vi "1 port_Parametric Calculations_MultiTest.vi"(0 "Port Measurements":T1, 2 "Specific Voltages":dbl[](array[numeric])=[32.0, 36.0], 11 "Error In":errorcluster) -> (4 "One_port_Parametric Calculated Values":T4, 15 "Error Out":errorcluster)   [LabVIEW 2013]
uses:
  Controls/Port Measurements.ctl
  Controls/1 port_Parametric Calculated Values.ctl
  Controls/Port Capacitance Parametric Calculations.ctl
  Controls/Port Voltage Parametric Calculations.ctl
  Controls/Port Resistance Parametric Calculations.ctl
  Controls/Resistance Array Calculated Values.ctl
  Controls/Individual User Inputs_MultiTest.ctl
  Controls/Test Selection.ctl
panel:
  in  "Tab Control":enum32{"Inputs", "Outputs"}(tab)
  in  "Selected Exp Settings":T2={"Floor_Sweep_Stop_V"=36.0, "Resistance Threshold"=1.0, "Floor_Sweep_Start_V"=36.0, "Floor_Sweep_Step_V"=1.0, "Roof_Sweep_Stop_V"=36.0, "Roof_Sweep_Start_V"=36.0, "Roof_Sweep_Step_V"=1.0, "Experiment Name"="", "Meas_Type"=[0, 2, 4]}
  # "Calculation Settings"
  # "Test Settings"
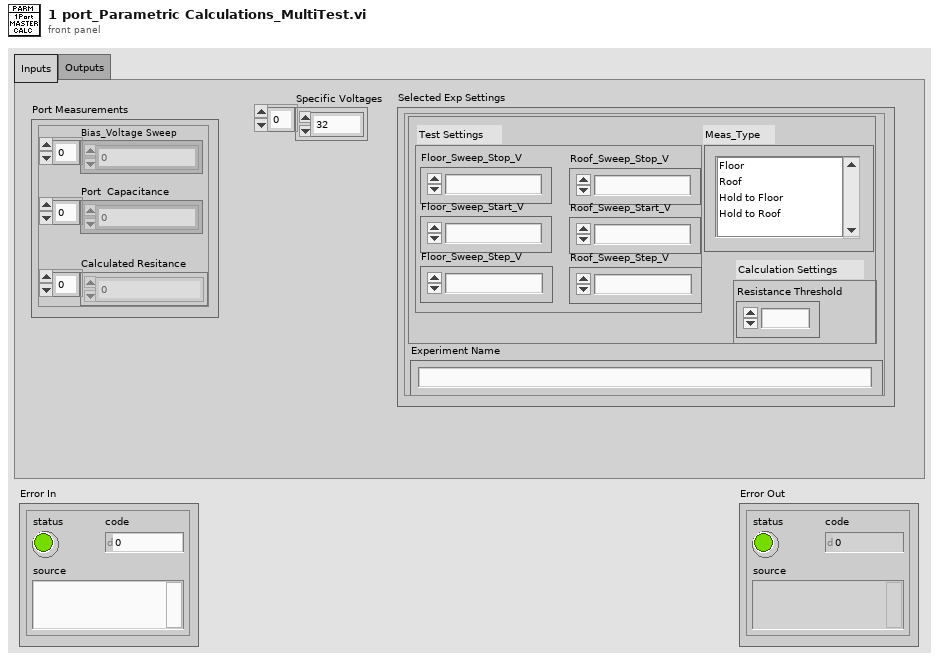
[diagram p1: front panel]
types:
  T1 = typedef "Port Measurements.ctl" = cluster{"Bias_Voltage Sweep":dbl[], "Port  Capacitance":dbl[], "Calculated Resitance":dbl[]}
  T2 = typedef "Individual User Inputs_MultiTest.ctl" = cluster{"Floor_Sweep_Stop_V":dbl, "Resistance Threshold":dbl, "Floor_Sweep_Start_V":dbl, "Floor_Sweep_Step_V":dbl, "Roof_Sweep_Stop_V":dbl, "Roof_Sweep_Start_V":dbl, "Roof_Sweep_Step_V":dbl, "Experiment Name":string, "Meas_Type":T3}
  T3 = typedef "Test Selection.ctl" = i32[]
  T4 = typedef "1 port_Parametric Calculated Values.ctl" = cluster{"Port Capacitance Parametic Calculations":T5, "Port Voltage Parametic Calculations":T6, "Port Resistance Parametric Calculations":T7, "Resistance Array Calc":T8}
  T5 = typedef "Port Capacitance Parametric Calculations.ctl" = cluster{"C_free":dbl, "C_vmax":dbl, "C_first":dbl, "C_last":dbl, "C_end":dbl, "Meas@Specific Voltages":dbl[]}
  T6 = typedef "Port Voltage Parametric Calculations.ctl" = cluster{"VPU_C":dbl, "VPU_Rel_C":dbl}
  T7 = typedef "Port Resistance Parametric Calculations.ctl" = cluster{"Rc_free":dbl, "Rc_first":dbl, "Rc_vmax":dbl, "Rc_last":dbl, "Rc_end":dbl, "VPD_R":dbl, "VPD_Rel_R":dbl}
  T8 = typedef "Resistance Array Calculated Values.ctl" = cluster{"RC@V":dbl[]}
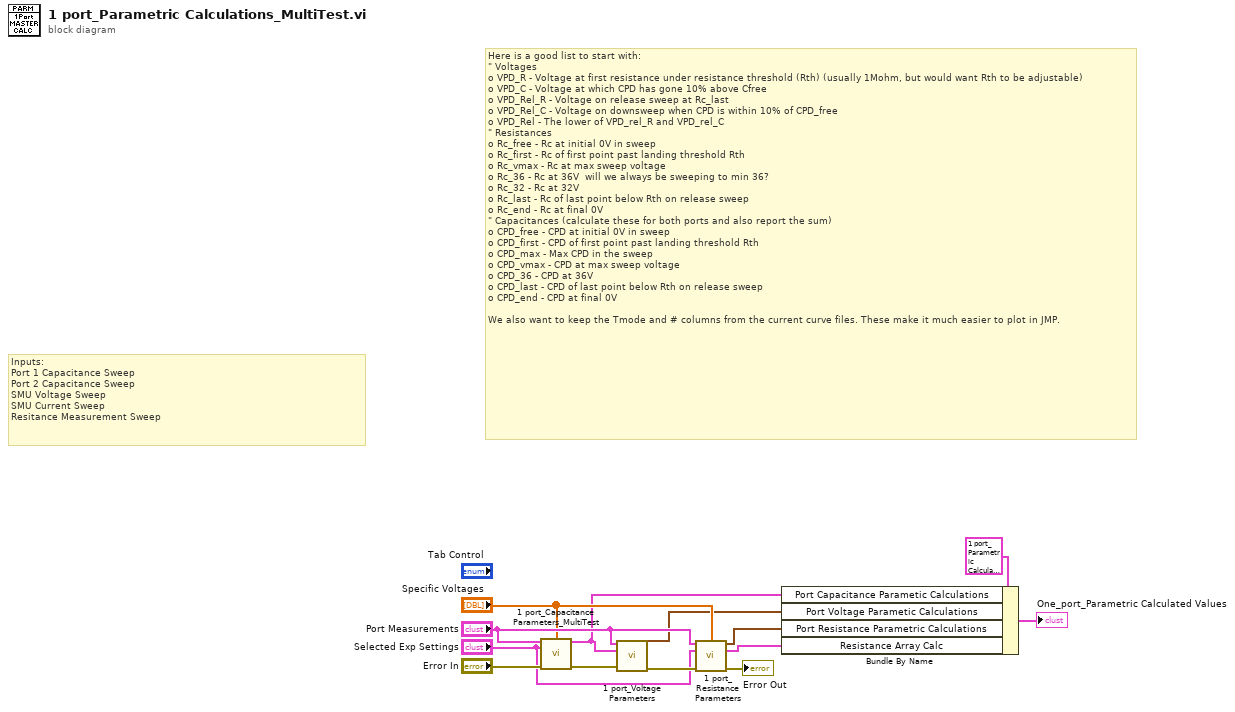
[diagram p0: block diagram]
diagram:
  # "Inputs:\nPort 1 Capacitance Sweep\nPort 2 Capacitance Sweep\nSMU Voltage Sweep\nSMU Current Sweep\nResitance Measurement Sweep"
  # "Here is a good list to start with:\n\"\tVoltages\no\tVPD_R - Voltage at first resistance under resistance threshold (Rth) (usually 1Mohm, but would want Rth to be adjustable)\no\tVPD_C - Voltage at which CPD has gone 10% above Cfree\no\tVPD_Rel_R - Voltage on release sweep at Rc_last\no\tVPD_Rel_C - Voltage on downsweep when CPD is within 10% of CPD_free\no\tVPD_Rel - The lower of VPD_rel_R and VPD_rel_C\n\"\tResistances\no\tRc_free - Rc at initial 0V in sweep\no\tRc_first - Rc of first point past landing threshold Rth \no\tRc_vmax - Rc at max sweep voltage\no\tRc_36 - Rc at 36V  will we always be sweeping to min 36?\no\tRc_32 - Rc at 32V\no\tRc_last - Rc of last point below Rth on release sweep\no\tRc_end - Rc at final 0V\n\"\tCapacitances (calculate these for both ports and also report the sum)\no\tCPD_free - CPD at initial 0V in sweep\no\tCPD_first - CPD of first point past landing threshold Rth \no\tCPD_max - Max CPD in the sweep\no\tCPD_vmax - CPD at max sweep voltage\no\tCPD_36 - CPD at 36V\no\tCPD_last - CPD of last point below Rth on release sweep\no\tCPD_end - CPD at final 0V\n \nWe also want to keep the Tmode and # columns from the current curve files. These make it much easier to plot in JMP."
  n1 = call "1 port_Capacitance Parameters_MultiTest.vi"("Port Measurements"="Port Measurements", "Specific Voltages"="Specific Voltages", "Selected Exp Settings"="Selected Exp Settings", "Error In"="Error In") -> ("Port Capacitance Parametic Calculations"=w6:T5, "Error Out"=w13:errorcluster)  [unwired: 10 in]
  n2 = call "1 port_Voltage Parameters.vi"("Port Measurements"="Port Measurements", "Port Parametic Calculations"=w6, "Error In"=w13) -> ("Port Voltage Parametic Calculations"=w5:T6, "Error Out"=w12:errorcluster)  [unwired: 11 in]
  n3 = call "1 port_Resistance Parameters.vi"("Port Measurements"="Port Measurements", "Specific Voltages 2"="Specific Voltages", "Selected Exp Settings"="Selected Exp Settings", "Error In"=w12) -> ("Port Resistance Parametric Calculations"=w4:T7, "Resistance Array Calc"=w3:T8, "Error Out"=→"Error Out":errorcluster)  [unwired: 9 in]
  n4 = Bundle By Name(cluster=T4 {"Port Capacitance Parametic Calculations"={"C_free"=0.0, "C_vmax"=0.0, "C_first"=0.0, "C_last"=0.0, "C_end"=0.0, "Meas@Specific Voltages"=[]}, "Port Voltage Parametic Calculations"={"VPU_C"=0.0, "VPU_Rel_C"=0.0}, "Port Resistance Parametric Calculations"={"Rc_free"=0.0, "Rc_first"=0.0, "Rc_vmax"=0.0, "Rc_last"=0.0, "Rc_end"=0.0, "VPD_R"=0.0, "VPD_Rel_R"=0.0}, "Resistance Array Calc"={"RC@V"=[]}} ("Parametric Calculated Values 2"), "Port Capacitance Parametic Calculations"=w6, "Port Voltage Parametic Calculations"=w5, "Port Resistance Parametric Calculations"=w4, "Resistance Array Calc"=w3) -> (→"One_port_Parametric Calculated Values":T4)
